vi "GetPrensentFrame.vi"(4 "database in":refnum<k21>="MLBevo_KCAN_KMatrix_V8", 5 "Cluster::":refnum<k21>, 7 "error in (no error)":errorcluster, 9 "New Frame Properties":T1={"Comment"="Tester_Present", "Default Payload"=[80], "Identifier"=62, "Name (Short)"="TstrPrsnt", "Payload Length"=1, "PDU_Mapping"=[], "CAN:Extended Identifier?"=FALSE, "CAN:Timing Type"=0, "CAN:Transmit Time"=0.1, "CAN:I/O Mode"=0} {"CAN:I/O Mode" items=["CAN 2.0", "CAN FD", "CAN FD+BRS"]; "Identifier" format="%.0x"; "CAN:Timing Type" items=["Cyclic Data", "Event Data", "Cyclic Remote", "Event Remote", "Cyclic/Event"]; "Default Payload" format="%.0x"}, 15 "frame name":string="Tester_Present") -> (24 "database out":refnum<k21>, 25 "target cluster out":refnum<k21>, 27 "error out":errorcluster={"status"=TRUE, "code"=-1074384540, "source"="Property Node (arg 6) in make tester present frame.vi \nProperty: PDU_Mapping"})   [LabVIEW 2018]
uses:
  <vilib>/xnet/xnet.llb/XNET Merge Copy Mode.ctl
  <vilib>/xnet/xnet.llb/XNET Database Create (Frame).vi
  <vilib>/xnet/xnet.llb/XNET Database Merge (Cluster).vi
  <resource>/objmgr/xnet.rc
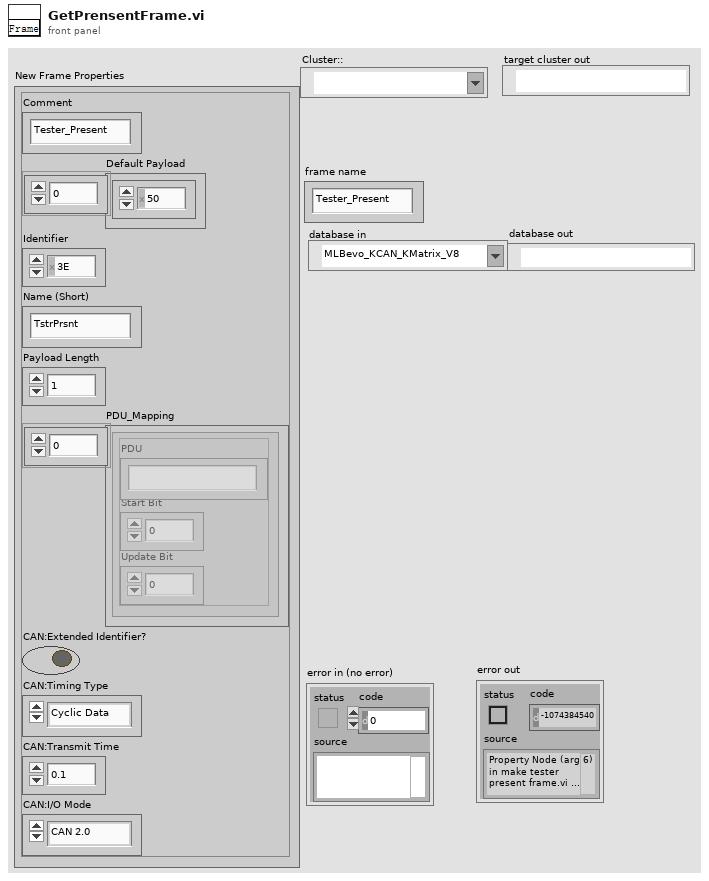
[diagram p1: front panel]
types:
  T1 = cluster{"Comment":string, "Default Payload":u8[], "Identifier":u32, "Name (Short)":string, "Payload Length":u32, "PDU_Mapping":cluster{"PDU":string, "Start Bit":u32, "Update Bit":i32}[], "CAN:Extended Identifier?":bool, "CAN:Timing Type":u32, "CAN:Transmit Time":dbl, "CAN:I/O Mode":u32}
  T2 = typedef "XNET Merge Copy Mode.ctl" = u32
  T3 = cluster{"PDU":string, "Start Bit":u32, "Update Bit":i32}[]
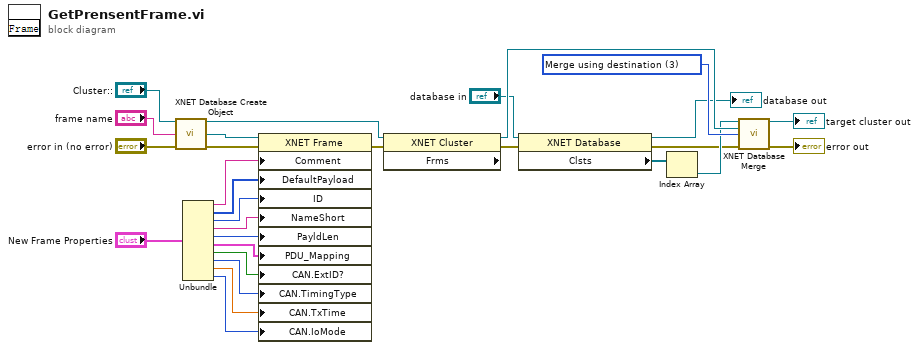
[diagram p0: block diagram]
diagram:
  w25 = T2 3 items=["Copy using source", "Copy using destination", "Merge using source", "Merge using destination"] ("copy mode")
  n1 = call-poly <vilib>:"XNET Database Create Object.vi"("cluster in"="Cluster::", "frame name"="frame name", "error in (no error)"="error in (no error)") -> ("cluster out"=w13:refnum<k21>, "frame out"=w27:refnum<k21>, "error out"=w26:errorcluster)  [unwired: 10 in]
  n2 = Unbundle("New Frame Properties") -> ("Comment"=w23:string, "Default Payload"=w22:u8[], "Identifier"=w21:u32, "Name (Short)"=w20:string, "Payload Length"=w19:u32, "PDU_Mapping"=w18:T3, "CAN:Extended Identifier?"=w17:bool, "CAN:Timing Type"=w16:u32, "CAN:Transmit Time"=w15:dbl, "CAN:I/O Mode"=w14:u32)
  n3 = property class="XNET Frame"(reference=w27, error in=w26, "Comment"=w23, "DefaultPayload"=w22, "ID"=w21, "NameShort"=w20, "PayldLen"=w19, "PDU_Mapping"=w18, "CAN.ExtID?"=w17, "CAN.TimingType"=w16, "CAN.TxTime"=w15, "CAN.IoMode"=w14) -> (error out=w12:errorcluster)  [unwired: 1 out]
  n4 = property class="XNET Cluster" props=["Frms"](reference=w13, error in=w12) -> (reference out=w11:refnum<k21>, error out=w7:errorcluster)  [unwired: 1 out]
  n5 = property class="XNET Database"(reference="database in", error in=w7) -> (reference out=→"database out":refnum<k21>, error out=w6:errorcluster, "Clsts"=w9:refnum<k21>[])
  n6 = Index Array(array=w9) -> (element=w8:refnum<k21>)  [unwired: 1 in]
  n7 = call-poly <vilib>:"XNET Database Merge.vi"("target cluster in"=w8, "source cluster"=w11, "copy mode"=w25, "error in (no error)"=w6) -> ("target cluster out"=→"target cluster out":refnum<k21>, "error out"=→"error out":errorcluster)  [unwired: 9 in, 1 out]
